vi "write all Array of U64s.vi"(8 "error in":errorcluster, 10 "values":cluster{"Array":u64[]}[](array[cluster]), 11 "data table in":T1) -> (0 "error out":errorcluster, 3 "data table out":T1)   [LabVIEW 2013, in "tag bus.lvlib" / "data table.lvlib"]
doc: "Replaces the entire set of values in the data table. If the size of the provided array does not match the array stored in the table, an error is thrown."
uses:
  data table.lvlib
  data table.ctl
  tag bus.lvlib
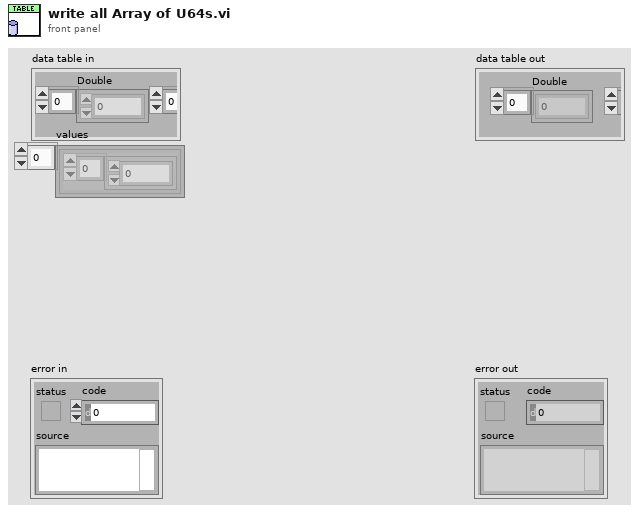
[diagram p1: front panel]
types:
  T1 = typedef "tag bus.lvlib/data table.lvlib/data table.ctl" = cluster{"Double":dbl[], "Single":sgl[], "I64":i64[], "I32":i32[], "I16":i16[], "I8":i8[], "U64":u64[], "U32":u32[], "U16":u16[], "U8":u8[], "Boolean":bool[], "String":string[], "Array of Double":cluster{"DBL Array":dbl[]}[], "Array of Single":cluster{"SGL Array":sgl[]}[], "Array of I64":cluster{"I64 Array":i64[]}[], "Array of I32":cluster{"I32 Array":i32[]}[], "Array of I16":cluster{"I16 Array":i16[]}[], "Array of I8":cluster{"I8 Array":i8[]}[], "Array of U64":cluster{"U64 Array":u64[]}[], "Array of U32":cluster{"U32 Array":u32[]}[], "Array of U16":cluster{"U16 Array":u16[]}[], "Array of U8":cluster{"U8 Array":u8[]}[], "Array of Boolean":cluster{"Boolean Array":bool[]}[], "Array of String":cluster{"String Array":string[]}[]}
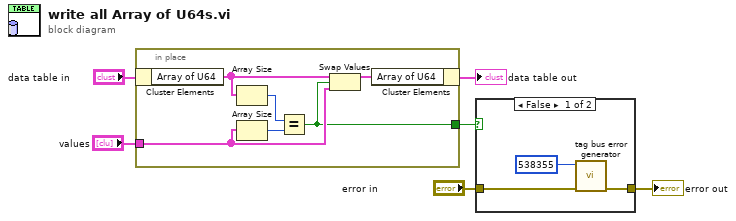
[diagram p0: block diagram]
diagram:
  n1 = in-place {
    in-place-border: "values" -> [w8]
    in-place-border: [w7] -> w3
    n2 = in-place-cluster #1("data table in") -> ("Array of U64"=w10:cluster{"U64 Array":u64[]}[])
    n3 = Array Size(array=w10) -> (size(s)=w12:i32)
    n4 = Array Size(array=w8) -> (size(s)=w11:i32)
    n5 = Equal?(x=w12, y=w11) -> (x = y?=w7:bool)
    n6 = Swap Values(12:w10, 13:w7, 14:w8) -> (1:w9:cluster{"U64 Array":u64[]}[])  [unwired: 1 out]
    n7 = in-place-cluster #1("Array of U64"=w9) -> (→"data table out":T1)
  }
  n8 = case shown="False" w3 {
    tunnel: [w15 w16] -> w2
    tunnel: "error in" -> [w14 w16]
    frame False {
      n9 = call "tag bus error generator.vi"("error in"=w14, "error code (0)"=538355) -> ("error out"=w15:errorcluster)  [unwired: 7 in]
    }
    frame True {
    }
  }
  "error out" <- w2
